vi "RFC5322 DateString to Timestamp.vi"(7 "RFC850|ANSI-C permissive?":bool, 8 "deprecated":bool=TRUE, 11 "RFC5322 String":string) -> (1 "valid?":bool, 2 "UTC Time Offset":T1=enum."UTC-00:00", 3 "Timestamp":timestamp)   [LabVIEW 2013]
uses:
  UTC Offsets -- enum.ctl
  <vilib>/Utility/miscctls.llb/LVDateTimeRec.ctl
  <vilib>/regexp/Match Regular Expression.xnode
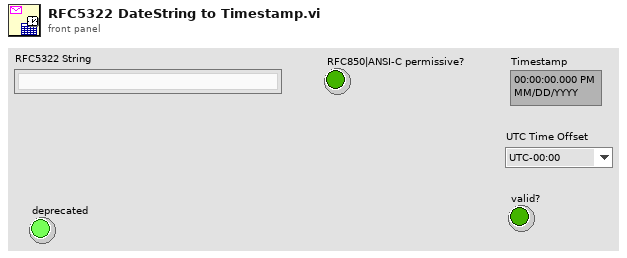
[diagram p1: front panel]
types:
  T1 = typedef "UTC Offsets -- enum.ctl" = enum16{"UTC-12:00", "UTC-11:00", "UTC-10:00", "UTC-09:30", "UTC-09:00", "UTC-08:00", "UTC-07:00", "UTC-06:00", "UTC-05:00", "UTC-04:00", "UTC-03:30", "UTC-03:00", "UTC-02:00", "UTC-01:00", "UTC-00:00", "UTC+00:00", "UTC+01:00", "UTC+02:00", "UTC+03:00", "UTC+03:30", "UTC+04:00", "UTC+04:30", "UTC+05:00", "UTC+05:30", "UTC+05:45", "UTC+06:00", "UTC+06:30", "UTC+07:00", "UTC+08:00", "UTC+08:45", "UTC+09:00", "UTC+09:30", "UTC+10:00", "UTC+10:30", "UTC+11:00", "UTC+12:00", "UTC+12:45", "UTC+13:00", "UTC+14:00"}
  T2 = typedef "LVDateTimeRec.ctl" = cluster{"fractional second":dbl, "second":i32, "minute":i32, "hour":i32, "day of month":i32, "month":i32, "year":i32, "day of week":i32, "day of year":i32, "DST":i32}
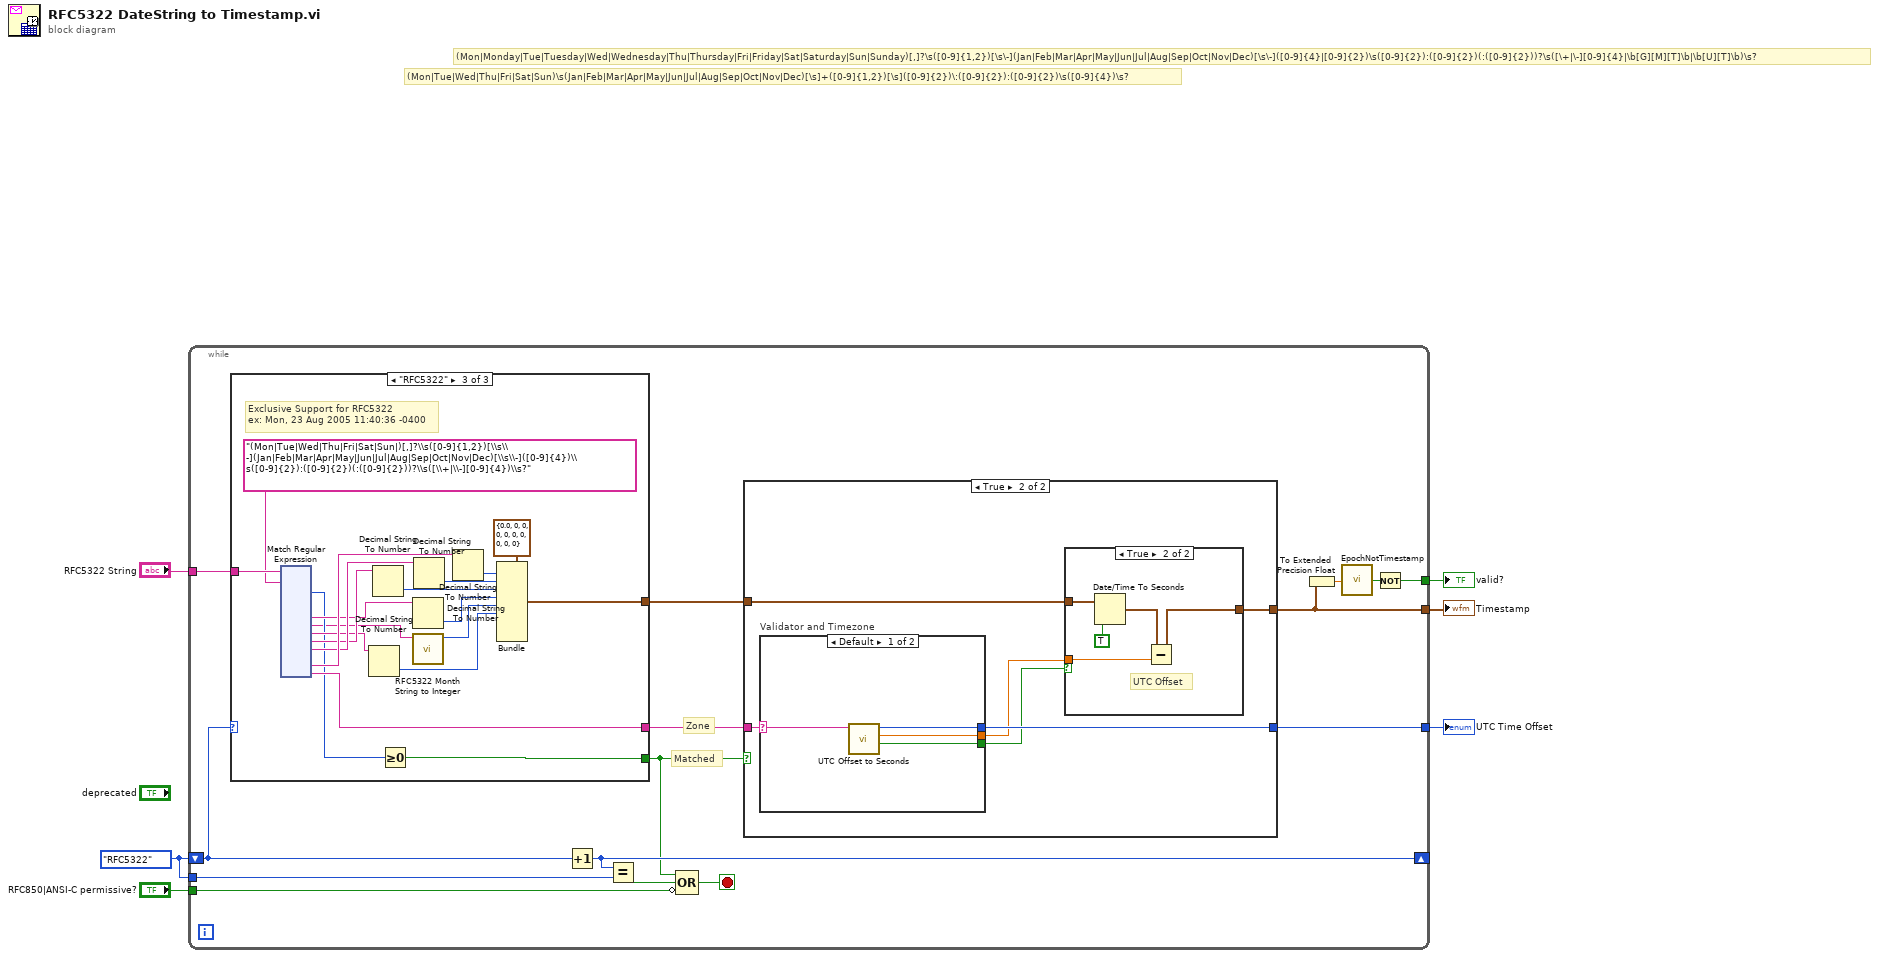
[diagram p0: block diagram]
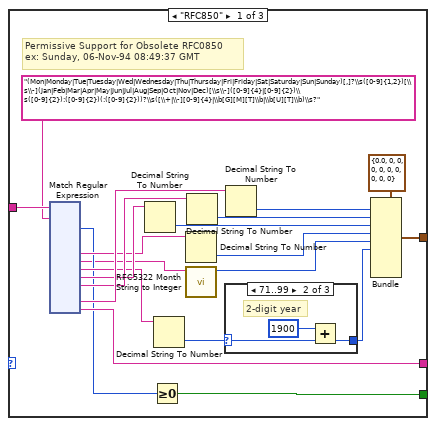
[diagram p2: hidden frame]
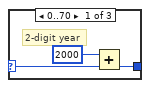
[diagram p3: hidden frame]
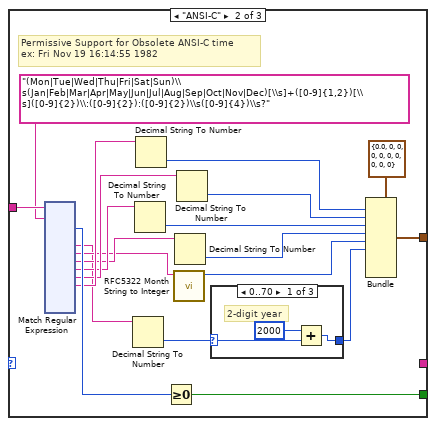
[diagram p5: hidden frame]
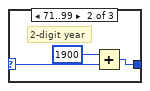
[diagram p6: hidden frame]
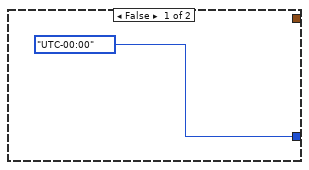
[diagram p8: hidden frame]
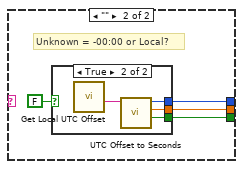
[diagram p9: hidden frame]
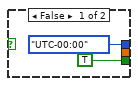
[diagram p10: hidden frame]
diagram:
  w2 = enum16{"RFC5322", "RFC850", "ANSI-C"}."RFC5322"
  # "(Mon|Tue|Wed|Thu|Fri|Sat|Sun)\\s(Jan|Feb|Mar|Apr|May|Jun|Jul|Aug|Sep|Oct|Nov|Dec)[\\s]+([0-9]{1,2})[\\s]([0-9]{2})\\:([0-9]{2}):([0-9]{2})\\s([0-9]{4})\\s?"
  # "(Mon|Monday|Tue|Tuesday|Wed|Wednesday|Thu|Thursday|Fri|Friday|Sat|Saturday|Sun|Sunday)[,]?\\s([0-9]{1,2})[\\s\\-](Jan|Feb|Mar|Apr|May|Jun|Jul|Aug|Sep|Oct|Nov|Dec)[\\s\\-]([0-9]{4}|[0-9]{2})\\s([0-9]{2}):([0-9]{2})(:([0-9]{2}))?\\s([\\+|\\-][0-9]{4}|\\b[G][M][T]\\b|\\b[U][T]\\b)\\s?"
  n1 = while {
    tunnel: [w8] -> w6
    tunnel: [w12] -> w5
    tunnel: [w19] -> w4
    tunnel: "RFC850|ANSI-C permissive?" -> [w17]
    shift-right: [w16] -> _
    shift-left: w2 -> [w13]
    tunnel: w2 -> [w14]
    tunnel: "RFC5322 String" -> [w11]
    stop <- w18 stop-if-true
    # "Zone"
    # "Matched"
    n2 = case shown="\"RFC5322\"" w13 {
      tunnel: w11 -> [w31 w185 w341]
      tunnel: [w30 w176 w328] -> w10
      tunnel: [w26 _ w327] -> w9
      tunnel: [w24 w183 w325] -> w7
      frame "RFC850" {
        # "Permissive Support for Obsolete RFC0850\nex: Sunday, 06-Nov-94 08:49:37 GMT"
        n3 = xnode "Match Regular Expression"("input string"=w31, "regular expression"="(Mon|Monday|Tue|Tuesday|Wed|Wednesday|Thu|Thursday|Fri|Friday|Sat|Saturday|Sun|Sunday)[,]?\\s([0-9]{1,2})[\\s\\-](Jan|Feb|Mar|Apr|May|Jun|Jul|Aug|Sep|Oct|Nov|Dec)[\\s\\-]([0-9]{4}|[0-9]{2})\\s([0-9]{2}):([0-9]{2})(:([0-9]{2}))?\\s([\\+|\\-][0-9]{4}|\\b[G][M][T]\\b|\\b[U][T]\\b)\\s?") -> ("offset past match"=w25:i32, "submatch 2"=w34:string, "submatch 3"=w23:string, "submatch 4"=w32:string, "submatch 5"=w36:string, "submatch 6"=w38:string, "submatch 8"=w40:string, "submatch 9"=w26:string)  [unwired: 4 in, 6 out]
        n4 = Decimal String To Number(string=w36) -> (number=w35:i32)  [unwired: 2 in, 1 out]
        n5 = Greater Or Equal To 0?(x=w25) -> (x >= 0?=w24:bool)
        n6 = Decimal String To Number(string=w32) -> (number=w28:i32)  [unwired: 2 in, 1 out]
        n7 = Decimal String To Number(string=w34) -> (number=w33:i32)  [unwired: 2 in, 1 out]
        n8 = call "RFC5322 Month String to Integer.vi"("Month (string)"=w23) -> ("Month (Number)"=w22:i32)  [unwired: 10 in]
        n9 = Decimal String To Number(string=w38) -> (number=w37:i32)  [unwired: 2 in, 1 out]
        n10 = case shown="71..99" w28 {
          selector: w28 -> [w44 w47 w48]
          tunnel: [w43 w46 w48] -> w27
          frame 0..70 {
            # "2-digit year"
            n11 = Add(x=2000, y=w44) -> (x+y=w43:i32)
          }
          frame 71..99 {
            # "2-digit year"
            n12 = Add(x=1900, y=w47) -> (x+y=w46:i32)
          }
          frame Default {
            # "4-digit year"
          }
        }
        n13 = Decimal String To Number(string=w40) -> (number=w39:i32)  [unwired: 2 in, 1 out]
        n14 = Bundle(cluster=T2 {"fractional second"=0.0, "second"=0, "minute"=0, "hour"=0, "day of month"=0, "month"=0, "year"=0, "day of week"=0, "day of year"=0, "DST"=0} ("date time rec"), "second"=w39, "minute"=w37, "hour"=w35, "day of month"=w33, "month"=w22, "year"=w27) -> (w30:T2)  [unwired: 4 in]
      }
      frame "ANSI-C" {
        # "Permissive Support for Obsolete ANSI-C time\nex: Fri Nov 19 16:14:55 1982"
        n15 = xnode "Match Regular Expression"("input string"=w185, "regular expression"="(Mon|Tue|Wed|Thu|Fri|Sat|Sun)\\s(Jan|Feb|Mar|Apr|May|Jun|Jul|Aug|Sep|Oct|Nov|Dec)[\\s]+([0-9]{1,2})[\\s]([0-9]{2})\\:([0-9]{2}):([0-9]{2})\\s([0-9]{4})\\s?") -> ("offset past match"=w184:i32, "submatch 1"=w177:string, "submatch 2"=w178:string, "submatch 3"=w179:string, "submatch 4"=w180:string, "submatch 5"=w181:string, "submatch 6"=w182:string)  [unwired: 4 in, 7 out]
        n16 = Decimal String To Number(string=w177) -> (number=w175:i32)  [unwired: 2 in, 1 out]
        n17 = Decimal String To Number(string=w180) -> (number=w188:i32)  [unwired: 2 in, 1 out]
        n18 = Decimal String To Number(string=w182) -> (number=w190:i32)  [unwired: 2 in, 1 out]
        n19 = Greater Or Equal To 0?(x=w184) -> (x >= 0?=w183:bool)
        n20 = call "RFC5322 Month String to Integer.vi"("Month (string)"=w178) -> ("Month (Number)"=w186:i32)  [unwired: 10 in]
        n21 = Decimal String To Number(string=w179) -> (number=w187:i32)  [unwired: 2 in, 1 out]
        n22 = Decimal String To Number(string=w181) -> (number=w189:i32)  [unwired: 2 in, 1 out]
        n23 = case shown="0..70" w175 {
          selector: w175 -> [w194 w197 w198]
          tunnel: [w193 w196 w198] -> w174
          frame 0..70 {
            # "2-digit year"
            n24 = Add(x=2000, y=w194) -> (x+y=w193:i32)
          }
          frame 71..99 {
            # "2-digit year"
            n25 = Add(x=1900, y=w197) -> (x+y=w196:i32)
          }
          frame Default {
            # "4-digit year"
          }
        }
        n26 = Bundle(cluster=T2 {"fractional second"=0.0, "second"=0, "minute"=0, "hour"=0, "day of month"=0, "month"=0, "year"=0, "day of week"=0, "day of year"=0, "DST"=0} ("date time rec"), "second"=w190, "minute"=w189, "hour"=w188, "day of month"=w187, "month"=w186, "year"=w174) -> (w176:T2)  [unwired: 4 in]
      }
      frame "RFC5322" {
        # "Exclusive Support for RFC5322 \nex: Mon, 23 Aug 2005 11:40:36 -0400"
        n27 = xnode "Match Regular Expression"("input string"=w341, "regular expression"="(Mon|Tue|Wed|Thu|Fri|Sat|Sun|)[,]?\\s([0-9]{1,2})[\\s\\-](Jan|Feb|Mar|Apr|May|Jun|Jul|Aug|Sep|Oct|Nov|Dec)[\\s\\-]([0-9]{4})\\s([0-9]{2}):([0-9]{2})(:([0-9]{2}))?\\s([\\+|\\-][0-9]{4})\\s?") -> ("offset past match"=w326:i32, "submatch 2"=w332:string, "submatch 3"=w324:string, "submatch 4"=w329:string, "submatch 5"=w334:string, "submatch 6"=w336:string, "submatch 8"=w338:string, "submatch 9"=w327:string)  [unwired: 4 in, 6 out]
        n28 = Decimal String To Number(string=w329) -> (number=w330:i32)  [unwired: 2 in, 1 out]
        n29 = Decimal String To Number(string=w334) -> (number=w333:i32)  [unwired: 2 in, 1 out]
        n30 = Greater Or Equal To 0?(x=w326) -> (x >= 0?=w325:bool)
        n31 = Decimal String To Number(string=w332) -> (number=w331:i32)  [unwired: 2 in, 1 out]
        n32 = call "RFC5322 Month String to Integer.vi"("Month (string)"=w324) -> ("Month (Number)"=w323:i32)  [unwired: 10 in]
        n33 = Decimal String To Number(string=w336) -> (number=w335:i32)  [unwired: 2 in, 1 out]
        n34 = Decimal String To Number(string=w338) -> (number=w337:i32)  [unwired: 2 in, 1 out]
        n35 = Bundle(cluster=T2 {"fractional second"=0.0, "second"=0, "minute"=0, "hour"=0, "day of month"=0, "month"=0, "year"=0, "day of week"=0, "day of year"=0, "DST"=0} ("date time rec"), "second"=w337, "minute"=w335, "hour"=w333, "day of month"=w331, "month"=w323, "year"=w330) -> (w328:T2)  [unwired: 4 in]
      }
    }
    n36 = Increment(x=w13) -> (x+1=w16:enum16{"RFC5322", "RFC850", "ANSI-C"})
    n37 = Equal?(x=w16, y=w14) -> (x = y?=w15:bool)
    n38 = Compound Arithmetic op=OR(w7, w15, invert w17) -> (w18:bool)
    n39 = case shown="True" w7 {
      tunnel: [_ w472] -> w19
      tunnel: [UTC_Offsets_--_enum."UTC-00:00" ("UTC Time Offset") w471] -> w12
      tunnel: w9 -> [_ w468]
      tunnel: w10 -> [_ w467]
      frame False {
      }
      frame True {
        n40 = case "Validator and Timezone" shown="Default" w468 {
          selector: w468 -> [w476 _]
          tunnel: [w473 w478] -> w471
          tunnel: [w474 w479] -> w469
          tunnel: [w475 w477] -> w470
          frame Default {
            n41 = call "UTC Offset to Seconds.vi"("UTC Offset String"=w476) -> ("Valid?"=w475:bool, "Offset (s)"=w474:ext, "UTC Offset"=w473:T1)  [unwired: 7 in, 1 out]
          }
          frame "" {
            # "Unknown = -00:00 or Local?"
            n42 = case shown="True" FALSE {
              tunnel: [_ w485] -> w479
              tunnel: [UTC_Offsets_--_enum."UTC-00:00" ("UTC Time Offset") w484] -> w478
              tunnel: [TRUE w483] -> w477
              frame False {
              }
              frame True {
                n43 = call "Get Local UTC Offset.vi"() -> ("UTC Offset String"=w486:string)  [unwired: 8 in, 3 out]
                n44 = call "UTC Offset to Seconds.vi"("UTC Offset String"=w486) -> ("Valid?"=w483:bool, "Offset (s)"=w485:ext, "UTC Offset"=w484:T1)  [unwired: 7 in, 1 out]
              }
            }
          }
        }
        n45 = case shown="True" w470 {
          tunnel: w467 -> [_ w490]
          tunnel: w469 -> [_ w489]
          tunnel: [_ w487] -> w472
          frame False {
          }
          frame True {
            # "UTC Offset"
            n46 = Date/Time To Seconds(1:TRUE ("is UTC (F)"), 2:w490) -> (0:w488:timestamp)
            n47 = Subtract(x=w488, y=w489) -> (x-y=w487:timestamp)
          }
        }
      }
    }
    n48 = To Extended Precision Float(1:w19) -> (0:w20:ext)
    n49 = call "EpochNotTimestamp.vi"("Epoch Time"=w20) -> ("Not a Timestamp?"=w21:bool)  [unwired: 8 in]
    n50 = Not(x=w21) -> (.not. x?=w8:bool)
  }
  "Timestamp" <- w4
  "valid?" <- w6
  "UTC Time Offset" <- w5
